vi "exp sim BAP2B.vi"() -> ()   [LabVIEW 2014]
doc: "exp sim BAP2F\n\nDisplays acquisition graph and an analysis graph which can be fine-tuned by the user. This then can export the fitting parameters into a .txt file and saved in an appropriate directory. \n\nSubvis Used:\nDamp Sine Fit BAP2b, Damp Sine Wave Gen\n\nBeverly Abadines\nPHY 350\nBAP2F"
uses:
  typedefs/measurment parameters.ctl
  typedefs/damped wave parameter cluster.ctl
  <vilib>/Utility/file.llb/Write To Spreadsheet File (DBL).vi
panel:
  in  "Stop":bool
  in  "Save Data":bool
  out "Data to Save":dbl[][](array[numeric])
  in  "Fitting Parameters":T1={"amplitude (V)"=8.0, "frequency (Hz)"=10000.0, "start phase (deg)"=45.0, "decay rate (1/sec)"=10000.0} {"decay rate (1/sec)" scale=0.0..20000.0; "start phase (deg)" scale=-180.0..180.0; "frequency (Hz)" scale=0.0..20000.0; "amplitude (V)" scale=0.0..10.0}
  out "Analysis Graph":cluster{dbl[], "time array out (s)":dbl[]}[](graph)
  out "Acquisition Graph":T2(graph)
  out "count":i32
  in  "Measurement Parameters":T3={"time step (s)"=1e-06, "N meas"=500, "N meas reps"=100}
  in  "Start":bool
  # "Simulated Experiment"
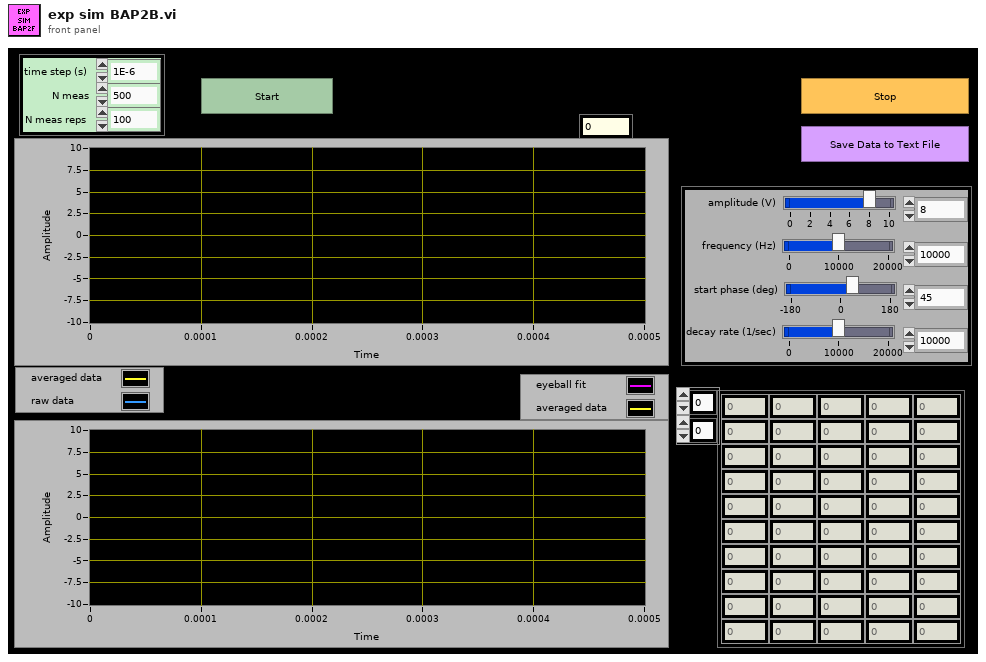
[diagram p1: front panel]
types:
  T1 = typedef "damped wave parameter cluster.ctl" = cluster{"amplitude (V)":dbl, "frequency (Hz)":dbl, "start phase (deg)":dbl, "decay rate (1/sec)":dbl}
  T2 = cluster{"time array (s)":dbl[], "voltage array (V)":dbl[]}[]
  T3 = typedef "measurment parameters.ctl" = cluster{"time step (s)":dbl, "N meas":i32, "N meas reps":i32}
  T4 = cluster{"time array (s)":dbl[], "voltage array (V)":dbl[]}
  T5 = cluster{"time array out (s)":dbl[], "voltage array out (V)":dbl[]}
  T6 = cluster{"time array out (s)":dbl[], "voltage array out (V)":dbl[]}[]
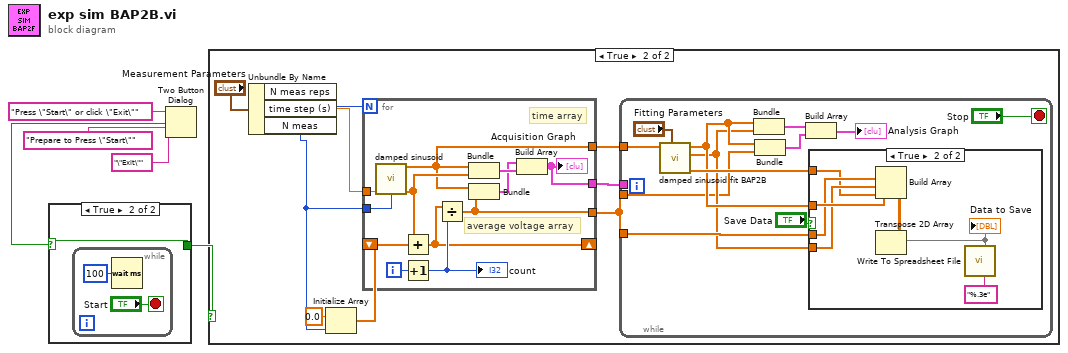
[diagram p0: block diagram]
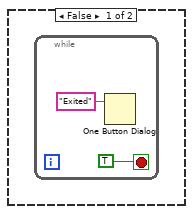
[diagram p3: hidden frame]
diagram:
  n1 = Two Button Dialog(message="Press \"Start\" or click \"Exit\"", 1:"\"Exit\"" ("F button name (\"Cancel\")"), 2:"Prepare to Press \"Start\"" ("T button name (\"OK\")")) -> (T button?=w2:bool)
  n2 = case shown="True" w2 {
    selector: w2 -> [w6 w7]
    tunnel: [w6 w7] -> w1
    frame False {
    }
    frame True {
      n3 = while {
        stop <- "Start" stop-if-true
        n4 = Wait (ms)(milliseconds to wait=u32 100) -> ()  [unwired: 1 out]
      }
    }
  }
  n5 = case shown="True" w1 {
    frame False {
      n6 = while {
        stop <- TRUE stop-if-true
        n7 = One Button Dialog(message="Exited") -> ()  [unwired: 1 in, 1 out]
      }
    }
    frame True {
      n8 = Unbundle By Name("Measurement Parameters") -> ("N meas reps"=w15:i32, "time step (s)"=w19:dbl, "N meas"=w16:i32)
      n9 = Initialize Array(0.0 ("element"), w16) -> (w18:dbl[])
      n10 = for {
        N: w15 -> [_]
        tunnel: w19 -> [w51]
        tunnel: w16 -> [w50]
        shift-right: [w45] -> _
        shift-left: w18 -> [w46]
        tunnel: [w42] -> w14
        tunnel: [w41] -> w12
        tunnel: [w40] -> w13
        i -> [w49]
        # "average voltage array"
        # "time array"
        n11 = call "damped sinusoid.vi"("time step (s)"=w51, "N meas"=w50) -> ("time array (s)"=w42:dbl[], "voltage array (V)"=w47:dbl[])  [unwired: 12 in]
        n12 = Add(x=w47, y=w46) -> (x+y=w45:dbl[])
        n13 = Increment(x=w49) -> (x+1=w48:i32)
        "count" <- w48
        n14 = Divide(x=w45, y=w48) -> (x/y=w41:dbl[])
        n15 = Bundle("time array (s)"=w42, "voltage array (V)"=w47) -> (w44:T4)  [unwired: 1 in]
        n16 = Bundle("time array (s)"=w42, w41) -> (w43:cluster{"time array (s)":dbl[], dbl[]})  [unwired: 1 in]
        n17 = Build Array(w43, w44) -> (w40:T2)
        "Acquisition Graph" <- w40
      }
      n18 = while {
        tunnel: w14 -> [w32]
        tunnel: w12 -> [w21]
        tunnel: w13 -> [_]
        tunnel: w12 -> [w26]
        stop <- "Stop" stop-if-true
        n19 = call "damped sinusoid fit BAP2B.vi"("fitting parameters"="Fitting Parameters", "time array in (s)"=w32) -> ("parameters array out"=w25:dbl[], "voltage array out (V)"=w22:dbl[], "time array out (s)"=w23:dbl[])  [unwired: 7 in]
        n20 = Bundle("time array out (s)"=w23, "voltage array out (V)"=w22) -> (w29:T5)  [unwired: 1 in]
        n21 = Bundle("time array out (s)"=w23, w21) -> (w24:cluster{"time array out (s)":dbl[], dbl[]})  [unwired: 1 in]
        n22 = Build Array(w29, w24) -> (→"Analysis Graph":T6)
        n23 = case shown="True" "Save Data" {
          tunnel: w23 -> [_ w38]
          tunnel: w26 -> [_ w37]
          tunnel: w22 -> [_ w36]
          tunnel: w25 -> [_ w35]
          frame False {
            # "Do Nothing"
          }
          frame True {
            n24 = Build Array(w38, w37, w36, w35) -> (w39:dbl[][])
            n25 = Transpose 2D Array(2D array=w39) -> (transposed array=w33:dbl[][])
            "Data to Save" <- w33
            n26 = call-poly <vilib>:"Write To Spreadsheet File.vi"("format (%.3f)"="%.3e", "2D data"=w33) -> ()  [unwired: 6 in, 1 out]
          }
        }
      }
    }
  }
